vi "三维表面.vi"() -> ()   [LabVIEW 2010]
uses:
  <vilib>/Platform/NI_3dgraph.lvlib
  <vilib>/Analysis/NI_AALBase.lvlib
panel:
  in  "三维曲面":refnum<k7>(container)
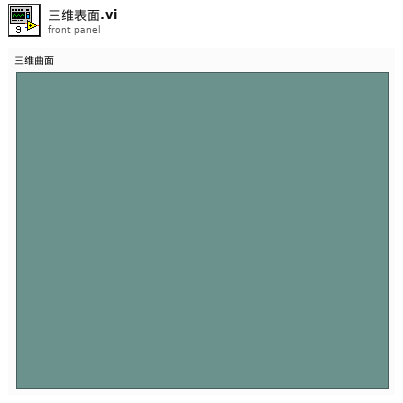
[diagram p1: front panel]
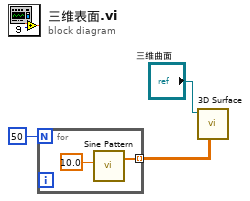
[diagram p0: block diagram]
diagram:
  n1 = for {
    N: 50 -> [_]
    tunnel: [w5] -> w1 mode=indexing
    n2 = call <vilib>:"Sine Pattern.vi"("amplitude"=10.0) -> ("Sinusoidal Pattern"=w5:dbl[])  [unwired: 3 in, 1 out]
  }
  n3 = call <vilib>:"3D Surface.vi"("z matrix"=w1, "3D graph"="三维曲面") -> ()  [unwired: 8 in, 2 out]
